vi "isresultok.vi"(10 "result":string) -> (2 "ok":bool)   [LabVIEW 2012]
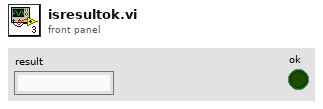
[diagram p1: front panel]
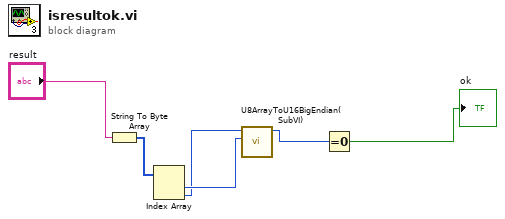
[diagram p0: block diagram]
diagram:
  n1 = String To Byte Array(string="result") -> (unsigned byte array=w6:u8[])
  n2 = Index Array(array=w6) -> (element #1=w5:u8, element #2=w4:u8)  [unwired: 2 in]
  n3 = call "U8ArrayToU16BigEndian(SubVI).vi"("Numeric 7"=w5, "Numeric 6"=w4) -> ("Numeric 9"=w2:u16)  [unwired: 9 in]
  n4 = Equal To 0?(x=w2) -> (x = 0?=→"ok":bool)
